vi "RNDUP.vi"(2 "X_ALIGN":i32=4, 3 "VAR":i32) -> (1 "RUDUP":i32)   [LabVIEW 2016]
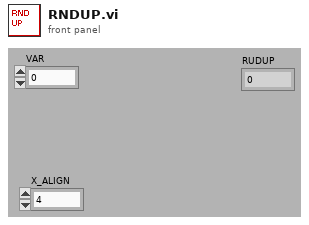
[diagram p1: front panel]
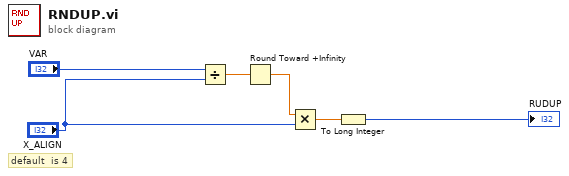
[diagram p0: block diagram]
diagram:
  # "default  is 4"
  n1 = Divide(x="VAR", y="X_ALIGN") -> (x/y=w4:dbl)
  n2 = Round Toward +Infinity(x=w4) -> (ceil(x): smallest int >= x=w5:dbl)
  n3 = Multiply(x=w5, y="X_ALIGN") -> (x*y=w3:dbl)
  n4 = To Long Integer(number=w3) -> (32bit integer=→"RUDUP":i32)
